vi "write_command.vi"(8 "error in (no error)":errorcluster, 10 "command (without terminating \"\\n\")":string, 11 "MH100301DMC in":refnum<class "StageMH100301DMC.lvclass">) -> (0 "error out":errorcluster, 2 "response out":string, 3 "MH100301DMC out":refnum<class "StageMH100301DMC.lvclass">)   [LabVIEW 2010, in "StageMH100301DMC.lvclass"]
uses:
  StageMH100301DMC.lvclass
  common/classes/ErrorController/ErrorController/ErrorController.lvclass
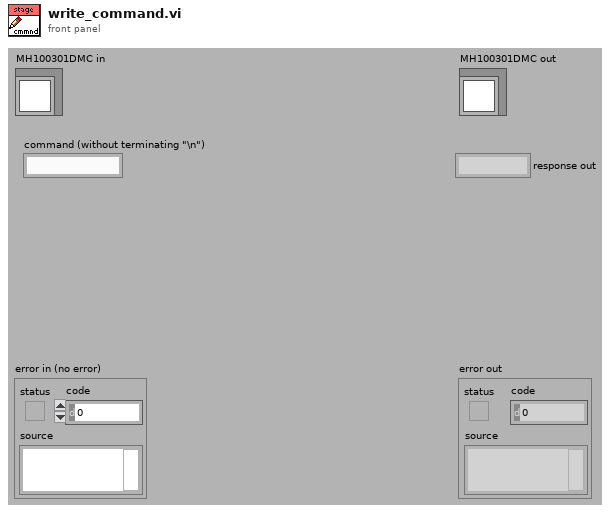
[diagram p1: front panel]
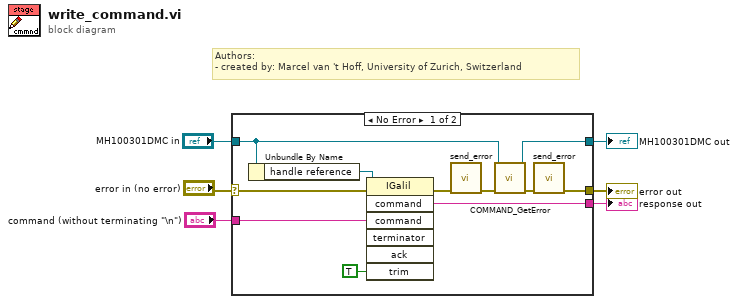
[diagram p0: block diagram]
diagram:
  # "Authors: \n- created by: Marcel van 't Hoff, University of Zurich, Switzerland"
  n1 = case shown="No Error" "error in (no error)" {
    selector: "error in (no error)" -> [w11 w19]
    tunnel: [w14 w19] -> w5
    tunnel: [w16 w18] -> w3
    tunnel: "MH100301DMC in" -> [w17 w18]
    tunnel: "command (without terminating \"\\n\")" -> [w10 _]
    tunnel: [w7 _] -> w1
    frame No Error {
      n2 = Unbundle By Name(w17) -> ("handle reference"=w12:refnum<k7>)
      n3 = invoke class="IGalil" method="command"(reference=w12, error in=w11, "command"=w10, "trim"=TRUE) -> (error out=w8:errorcluster, "command"=w7:string)  [unwired: 3 in, 5 out]
      n4 = call "send_error.vi"("error in (no error)"=w8) -> ("error out"=w13:errorcluster)  [unwired: 10 in]
      n5 = call-dynamic "COMMAND_GetError.vi"("error in (no error)"=w13, "StageMH100301DMC in"=w17) -> ("error out"=w15:errorcluster, "StageMH100301DMC out"=w16:refnum<class "StageMH100301DMC.lvclass">)  [unwired: 8 in]
      n6 = call "send_error.vi"("error in (no error)"=w15) -> ("error out"=w14:errorcluster)  [unwired: 10 in]
    }
    frame Error {
    }
  }
  "error out" <- w5
  "MH100301DMC out" <- w3
  "response out" <- w1
